vi "Voltage - Continuous Output.vi"() -> ()   [LabVIEW 2012]
doc: "This example demonstrates how to continuously re-generate analog output data from a buffer in your computer's memory.\n\nRefer to your device documentation for pinouts and hardware capabilities."
uses:
  <vilib>/DAQmx/write.llb/DAQmx Write (Analog 1D Wfm NChan NSamp).vi
  <vilib>/DAQmx/create/channels.llb/DAQmx Create Channel (AO-Voltage-Basic).vi
  <vilib>/DAQmx/configure/timing.llb/DAQmx Timing (Sample Clock).vi
  <vilib>/DAQmx/configure/trigger.llb/DAQmx Start Trigger (Digital Edge).vi
  <vilib>/DAQmx/configure/trigger.llb/DAQmx Start Trigger (Analog Edge).vi
  <vilib>/DAQmx/miscellaneous.llb/DAQmx Fill In Error Info.vi
  <resource>/objmgr/daqmx.rc
  <vilib>/measure/NI_MABase.lvlib
panel:
  in  "Output Array":T1(array[cluster])=[{"Waveform Type"=0, "Amplitude"=1.0, "Frequency"=10.0}] {"Frequency" format="%0.2p"; "Amplitude" format="%0.2p"; "Waveform Type" items=["Sine Wave", "Triangle Wave", "Square Wave", "Sawtooth Wave"]}
  in  "Number of Samples":i32=1000
  in  "Trigger Type":T2(tab)
  in  "Edge":i32(ring)=10280 items=["Rising"=10280, "Falling"=10171]
  in  "Digital Trigger Source":tag
  in  "Level (V)":dbl format="%0.2f"
  in  "Hysteresis (V)":dbl
  in  "Slope":i32(ring)=10280 items=["Rising"=10280, "Falling"=10171]
  in  "Analog Trigger Source":string="APFI0"
  in  "Pause When":i32(ring)=10192 items=["High"=10192, "Low"=10214]
  in  "Pause Trigger Source":tag
  in  "Stop":bool
  out "Waveform Graph":waveform(dbl)[](graph)=[{"t0"=timestamp(0 s since 1904-01-01), "dt"=0.001, "Y"=[]}]
  in  "Sample Rate":dbl=1000.0
  in  "Sample Clock Source":tag="OnboardClock"
  in  "Max Voltage":dbl=5.0
  in  "Min Voltage":dbl=-5.0
  in  "Physical Channel(s)":tag="Dev1/ao0"
  out "Actual Sample Rate":dbl=1000.0 format="%0.2f"
  # "Channel Settings"
  # "Output"
  # "Timing and Buffer Settings"
  # "Waveform Settings"
  # "Trigger Settings"
  # "The number of elements in the waveform array\nmust equal the number of channels in the task."
  # "To configure and use a start trigger you must have the necessary tab selected above.  Not all hardware supports triggering--refer to your device documentation for more info."
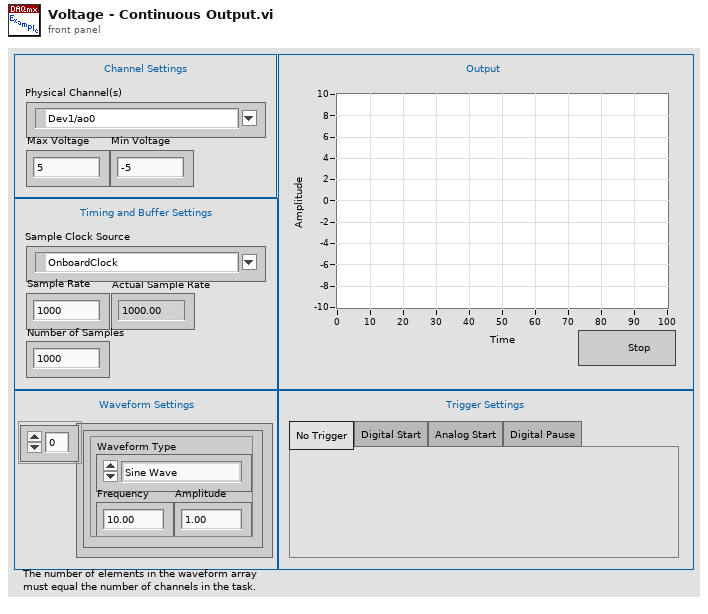
[diagram p1: front panel]
types:
  T1 = cluster{"Waveform Type":u16, "Amplitude":dbl, "Frequency":dbl}[]
  T2 = enum32{"No Trigger", "Digital Start", "Analog Start", "Digital Pause"}
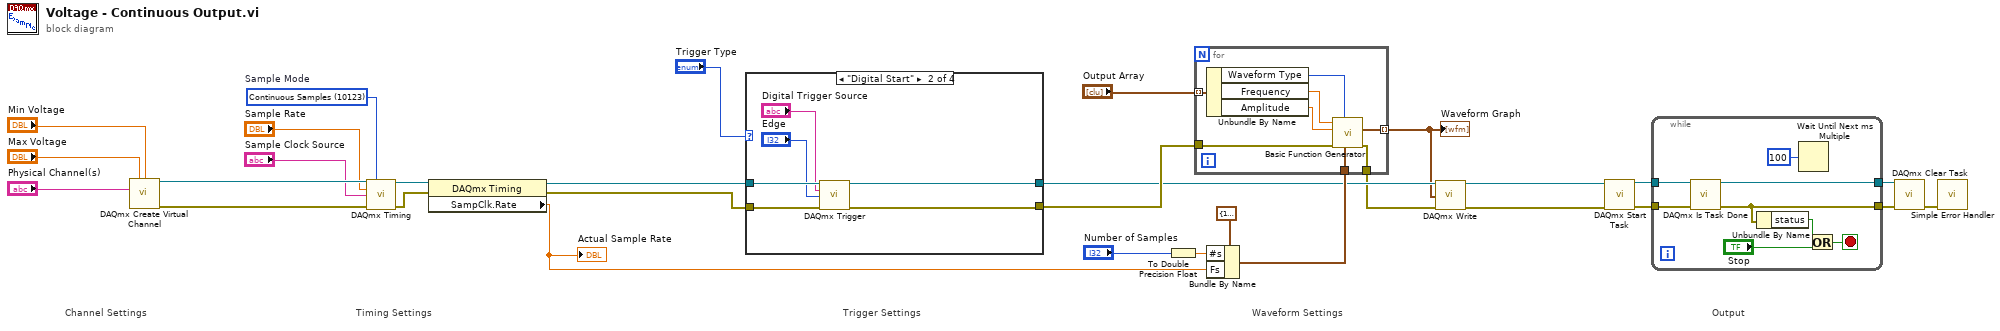
[diagram p0: block diagram]
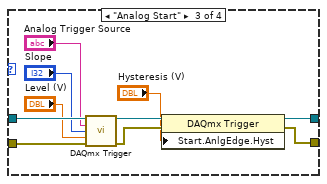
[diagram p3: hidden frame]
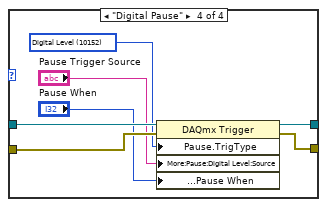
[diagram p4: hidden frame]
diagram:
  w28 = 10123 items=["Finite Samples"=10178, "Continuous Samples"=10123, "Hardware Timed Single Point"=12522]  # Sample Mode
  # "Output"
  # "Trigger Settings"
  # "Waveform Settings"
  # "Timing Settings"
  # "Channel Settings"
  n1 = call-poly <vilib>:"DAQmx Create Virtual Channel.vi"("maximum value"="Max Voltage", "minimum value"="Min Voltage", "physical channels"="Physical Channel(s)") -> ("task out"=w26:refnum<k21>, "error out"=w27:errorcluster)  [unwired: 11 in]
  n2 = call-poly <vilib>:"DAQmx Timing.vi"("task/channels in"=w26, "sample mode"=w28, "rate"="Sample Rate", "source"="Sample Clock Source", "error in"=w27) -> ("task out"=w30:refnum<k21>, "error out"=w29:errorcluster)  [unwired: 9 in]
  n3 = property class="DAQmx Timing"(reference=w30, error in=w29) -> (reference out=w14:refnum<k21>, error out=w13:errorcluster, "SampClk.Rate"=w10:dbl)
  "Actual Sample Rate" <- w10
  n4 = case shown="\"Digital Start\"" "Trigger Type" {
    tunnel: w14 -> [w32 w38 w48 w55]
    tunnel: w13 -> [w31 w37 w47 w52]
    tunnel: [w32 w36 w45 w54] -> w8
    tunnel: [w31 w35 w44 w53] -> w12
    frame "No Trigger", Default {
    }
    frame "Digital Start" {
      n5 = call-poly <vilib>:"DAQmx Trigger.vi"("task/channels in"=w38, "source"="Digital Trigger Source", "edge"="Edge", "error in"=w37) -> ("task out"=w36:refnum<k21>, "error out"=w35:errorcluster)  [unwired: 10 in]
    }
    frame "Analog Start" {
      n6 = call-poly <vilib>:"DAQmx Trigger.vi"("task/channels in"=w48, "source"="Analog Trigger Source", "slope"="Slope", "level"="Level (V)", "error in"=w47) -> ("task out"=w43:refnum<k21>, "error out"=w42:errorcluster)  [unwired: 9 in]
      n7 = property class="DAQmx Trigger"(reference=w43, error in=w42, "Start.AnlgEdge.Hyst"="Hysteresis (V)") -> (reference out=w45:refnum<k21>, error out=w44:errorcluster)
    }
    frame "Digital Pause" {
      w51 = 10152 items=["Analog Level"=10101, "Analog Window"=10103, "Digital Level"=10152, "Digital Pattern"=10398, "None"=10230] ("Pause.TrigType")
      n8 = property class="DAQmx Trigger"(reference=w55, error in=w52, "Pause.TrigType"=w51, "More:Pause:Digital Level:Source"="Pause Trigger Source", "More:Pause:Digital Level:Pause When"="Pause When") -> (reference out=w54:refnum<k21>, error out=w53:errorcluster)
    }
  }
  n9 = To Double Precision Float(number="Number of Samples") -> (double precision float=w2:dbl)
  n10 = Bundle By Name(cluster=cluster{"Fs":dbl, "#s":dbl} {"Fs"=1000.0, "#s"=1000.0} ("sampling info"), "#s"=w2, "Fs"=w10) -> (w9:cluster{"Fs":dbl, "#s":dbl})
  n11 = for {
    tunnel: w12 -> [w63]
    tunnel: w9 -> [w62]
    tunnel: [w61] -> w5
    tunnel: "Output Array" -> [w60] mode=indexing
    tunnel: [w56] -> w3 mode=indexing
    n12 = Unbundle By Name(w60) -> ("Waveform Type"=w59:u16, "Frequency"=w58:dbl, "Amplitude"=w57:dbl)
    n13 = call <vilib>:"Basic Function Generator.vi"("sampling info"=w62, "signal type"=w59, "error in (no error)"=w63, "amplitude"=w57, "frequency"=w58) -> ("error out"=w61:errorcluster, "signal out"=w56:waveform(dbl))  [unwired: 4 in, 1 out]
  }
  "Waveform Graph" <- w3
  n14 = call-poly <vilib>:"DAQmx Write.vi"("task/channels in"=w8, "data"=w3, "error in"=w5) -> ("task out"=w7:refnum<k21>, "error out"=w6:errorcluster)  [unwired: 10 in, 1 out]
  n15 = call <vilib>:"DAQmx Start Task.vi"("task/channels in"=w7, "error in"=w6) -> ("task out"=w25:refnum<k21>, "error out"=w24:errorcluster)  [unwired: 12 in]
  n16 = while {
    tunnel: w25 -> [w71]
    tunnel: w24 -> [w70]
    tunnel: [w67] -> w22
    tunnel: [w68] -> w23
    stop <- w69 stop-if-true
    n17 = call <vilib>:"DAQmx Is Task Done.vi"("task/channels in"=w71, "error in"=w70) -> ("task out"=w68:refnum<k21>, "error out"=w67:errorcluster)  [unwired: 11 in, 1 out]
    n18 = Unbundle By Name(w67) -> ("status"=w66:bool)
    n19 = Wait Until Next ms Multiple(millisecond multiple=u32 100) -> ()  [unwired: 1 out]
    n20 = Or(x=w66, y="Stop") -> (x .or. y?=w69:bool)
  }
  n21 = call <vilib>:"DAQmx Clear Task.vi"("task in"=w23, "error in"=w22) -> ("error out"=w21:errorcluster)  [unwired: 13 in]
  n22 = call <vilib>:"Simple Error Handler.vi"("error in (no error)"=w21) -> ()  [unwired: 4 in, 5 out]
